vi "SeqGet.vi"(8 "error in (no error)":errorcluster, 11 "Sequence in":refnum<class "Sequence.lvclass">) -> (0 "error out":errorcluster, 1 "Tag":string, 2 "Cohorts":refnum<class "Cohort.lvclass">[](array[class]), 3 "Sequence out":refnum<class "Sequence.lvclass">)   [LabVIEW 2012, in "Sequence.lvclass"]
uses:
  Sequence.lvclass
  Cohort.lvclass
  Sequence.lvclass/Sequence.ctl
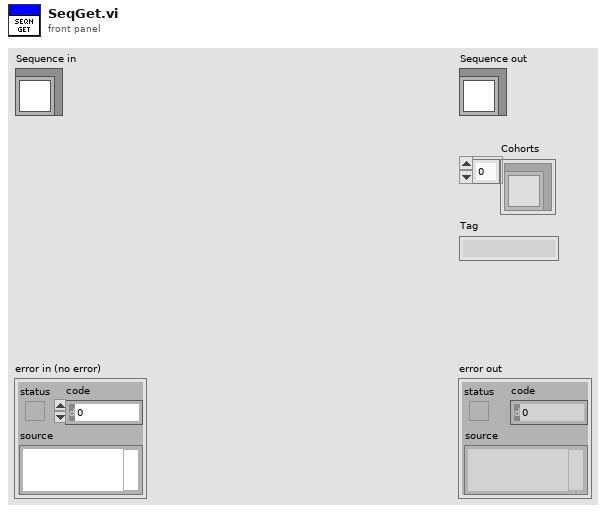
[diagram p1: front panel]
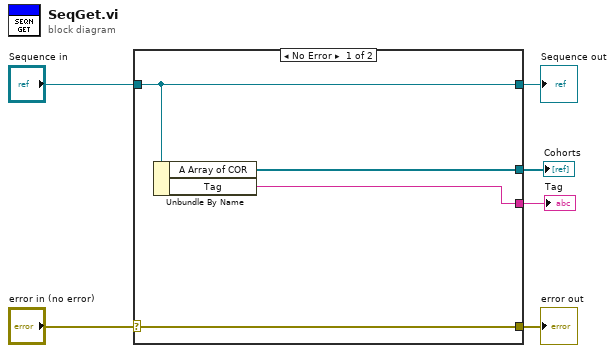
[diagram p0: block diagram]
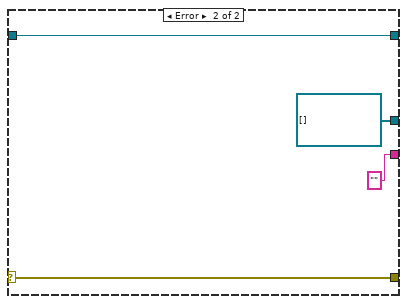
[diagram p2: hidden frame]
diagram:
  n1 = case shown="No Error" "error in (no error)" {
    selector: "error in (no error)" -> [w10 w13]
    tunnel: [w10 w13] -> w5
    tunnel: [w9 w14] -> w3
    tunnel: "Sequence in" -> [w9 w14]
    tunnel: [w8 refnum<class "Cohort.lvclass">[] [] ("Sequence")] -> w2
    tunnel: [w7 "" ("Tag")] -> w1
    frame No Error {
      n2 = Unbundle By Name(w9) -> ("A Array of COR"=w8:refnum<class "Cohort.lvclass">[], "Tag"=w7:string)
    }
    frame Error {
    }
  }
  "error out" <- w5
  "Sequence out" <- w3
  "Cohorts" <- w2
  "Tag" <- w1
